vi "Tosca-Initialize IPC.vi"() -> (4 "IPC":T1, 8 "Event Registration Refnum":refnum<event-registration>, 15 "error out":errorcluster)   [LabVIEW 2020]
uses:
  Tosca-IPC.ctl
  Classes/Parameters/Parameters.lvclass
  Digital Input VIs/Tosca-DI Queue Data.ctl
  Digital Input VIs/Tosca-Input Event.ctl
  Digital Input VIs/Tosca-Input Criterion.ctl
  epl-vi-lib/Utility VIs/Type Defs/Logic State.ctl
  Typedefs/Tosca-Accumulator.ctl
  Typedefs/Tosca-State AODO.ctl
  Typedefs/Tosca-AO Runtime.ctl
  Typedefs/Tosca-DO Runtime.ctl
  epl-vi-lib/Signal Synthesis VIs/4th Generation/Classes/SignalManager/SignalManager.lvclass
  Typedefs/Tosca-Synapse Start Data.ctl
  Tosca-Message.ctl
  Tosca-Message Action.ctl
  Typedefs/Tosca-Thread Type.ctl
  Imaging VIs/Tosca-2P-Notifier Data.ctl
  Typedefs/Tosca-MATLAB Queue Data.ctl
  Visual Stim VIs/Tosca-Grating.ctl
  Visual Stim VIs/Tosca-Grating Type.ctl
  Typedefs/Tosca-File IO Notification.ctl
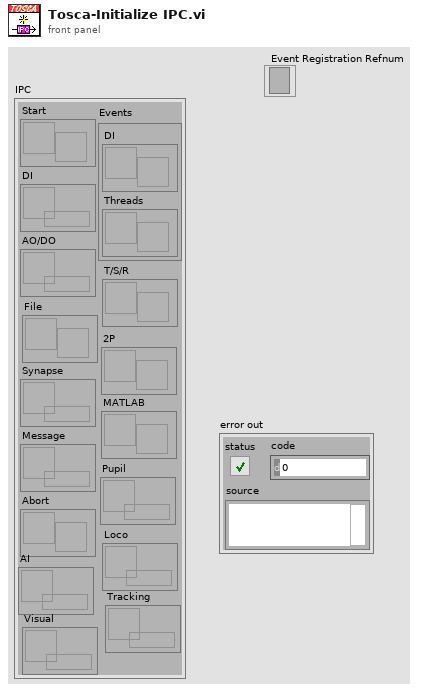
[diagram p1: front panel]
types:
  T1 = typedef "Tosca-IPC.ctl" = cluster{"Start":refnum<notifier>, "DI":refnum<queue>, "AO/DO":refnum<queue>, "Synapse":refnum<queue>, "Message":refnum<queue>, "Abort":refnum<notifier>, "Events":cluster{"DI":refnum<user-event>, "Threads ":refnum<user-event>}, "T/S/R":refnum<notifier>, "2P":refnum<notifier>, "MATLAB":refnum<notifier>, "Pupil":refnum<queue>, "Loco":refnum<queue>, "AI":refnum<queue>, "Tracking":refnum<queue>, "Visual":refnum<queue>, "File":refnum<notifier>}
  T2 = typedef "Tosca-Synapse Start Data.ctl" = cluster{"Path":path, "Codes":string, "retrieve":bool}
  T3 = typedef "Tosca-Grating.ctl" = cluster{"Type":T4, "Orientation (deg)":dbl, "Spatial frequency (cpd)":dbl, "Velocity (Hz)":dbl, "Contrast":dbl, "Background intensity":dbl, "Duration (ms)":dbl, "Phase (cycles)":dbl}
  T4 = typedef "Tosca-Grating Type.ctl" = enum16{"OFF", "Square", "Sine"}
  T5 = typedef "Tosca-MATLAB Queue Data.ctl" = cluster{"MATLAB function":path, "Datafile":path}
  T6 = typedef "Tosca-2P-Notifier Data.ctl" = cluster{"Start":bool}
  T7 = typedef "Tosca-Thread Type.ctl" = enum16{"None", "AODO", "Masker", "ET", "Imaging", "Pupil", "AI", "DI", "Camera", "TTL out", "Loco", "Visual"}
  T8 = typedef "Tosca-Message.ctl" = cluster{"Action":T9, "Time":u32, "State":i32, "Events":bool[], "Error":errorcluster}
  T9 = typedef "Tosca-Message Action.ctl" = enum16{"None", "Update", "Events", "Timeout", "Error", "Abort"}
  T10 = typedef "Tosca-File IO Notification.ctl" = cluster{"Operation":enum16{"Start", "Update", "Finish"}, "Filestem":string}
  T11 = typedef "Tosca-DI Queue Data.ctl" = cluster{"Action":enum16{"Stop", "Preview", "Run"}, "Input Events":T12[]}
  T12 = typedef "Tosca-Input Event.ctl" = cluster{"Name":string, "Criteria":T13[], "Operators":enum16{"AND", "OR"}[], "Accumulator":T15}
  T13 = typedef "Tosca-Input Criterion.ctl" = cluster{"DigInput":i32, "State":T14, "Time (ms)":i32, "Name":string}
  T14 = typedef "Logic State.ctl" = enum16{"Low", "High", "Rising", "Falling"}
  T15 = typedef "Tosca-Accumulator.ctl" = cluster{"active":bool, "N":i32, "T":dbl, "Imax":dbl, "latency":dbl}
  T16 = typedef "Tosca-State AODO.ctl" = cluster{"Name":string, "T (s)":dbl, "First AO":dbl[][], "frames/rep":i32, "finish?":bool, "Nrep":i32, "AO":T17, "DO":T18, "immediate":bool, "First DO":bool[][], "SigMan":refnum<class "SignalManager.lvclass">}
  T17 = typedef "Tosca-AO Runtime.ctl" = cluster{"Fs (Hz)":dbl, "pts/frame":i32, "pts/rep":i32, "ramp off":bool[], "fade out":dbl[][]}
  T18 = typedef "Tosca-DO Runtime.ctl" = cluster{"Fs (Hz)":dbl, "pts/frame":i32, "pts/rep":i32, "Rep":i32, "State":i32, "Trial":i32, "Frame":i32, "frOut":bool[], "Nchan":i32}
  T19 = cluster{"DI Thread State":refnum<user-event>, "Thread State":refnum<user-event>}
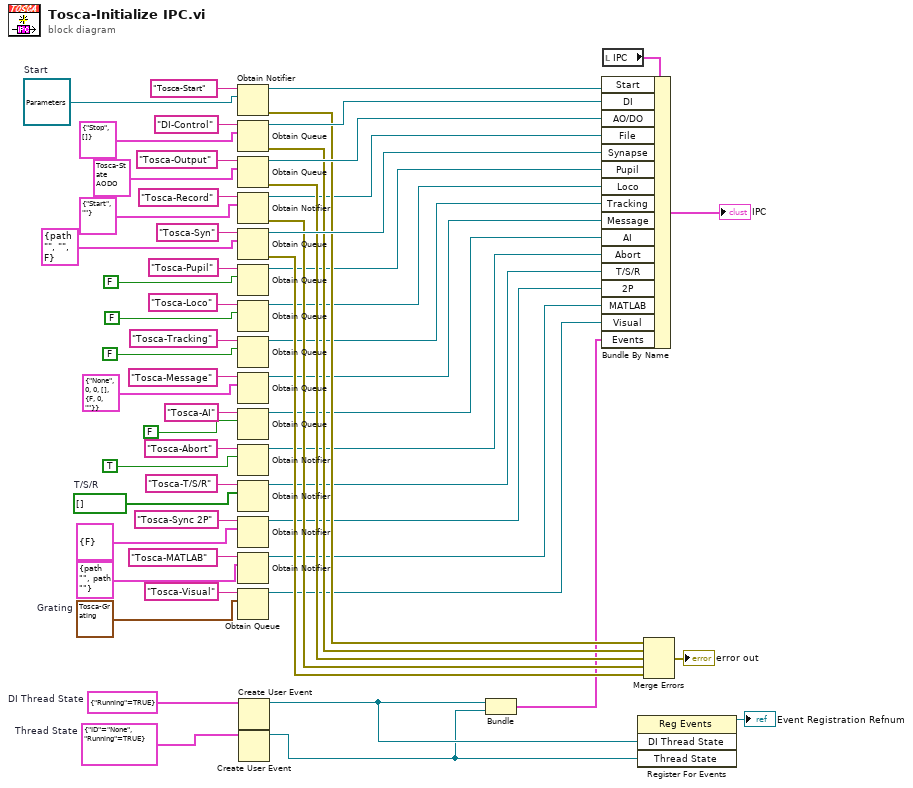
[diagram p0: block diagram]
diagram:
  w2 = refnum<class "Parameters.lvclass"> refnum  # Start
  w5 = T3 {"Type"=enum."OFF", "Orientation (deg)"=0.0, "Spatial frequency (cpd)"=0.0, "Velocity (Hz)"=0.0, "Contrast"=0.0, "Background intensity"=0.0, "Duration (ms)"=0.0, "Phase (cycles)"=0.0}  # Grating
  w26 = bool[] []  # T/S/R
  w31 = cluster{"ID":T7, "Running":bool} {"ID"=enum."None", "Running"=TRUE}  # Thread State
  w38 = cluster{"Running":bool} {"Running"=TRUE}  # DI Thread State
  n1 = Obtain Notifier(name (unnamed)="Tosca-Start" ("Start"), notification data type=w2) -> (notifier out=w53:refnum<notifier>, error out=w48:errorcluster)  [unwired: 2 in, 1 out]
  n2 = Obtain Queue(name (unnamed)="DI-Control", element data type=T11 {"Action"=enum."Stop", "Input Events"=[]} ("Cluster")) -> (queue out=w52:refnum<queue>, error out=w47:errorcluster)  [unwired: 3 in, 1 out]
  n3 = Obtain Queue(name (unnamed)="Tosca-Output", element data type=T16 {"Name"="", "T (s)"=0.0, "First AO"=[], "frames/rep"=0, "finish?"=FALSE, "Nrep"=0, "AO"={"Fs (Hz)"=0.0, "pts/frame"=0, "pts/rep"=0, "ramp off"=[], "fade out"=[]}, "DO"={"Fs (Hz)"=0.0, "pts/frame"=0, "pts/rep"=0, "Rep"=0, "State"=0, "Trial"=0, "Frame"=0, "frOut"=[], "Nchan"=0}, "immediate"=FALSE, "First DO"=[], "SigMan"=refnum} ("Output State Data")) -> (queue out=w51:refnum<queue>, error out=w46:errorcluster)  [unwired: 3 in, 1 out]
  n4 = Obtain Notifier(name (unnamed)="Tosca-Record" ("Start"), notification data type=T10 {"Operation"=enum."Start", "Filestem"=""} ("Data")) -> (notifier out=w39:refnum<notifier>, error out=w40:errorcluster)  [unwired: 2 in, 1 out]
  n5 = Obtain Queue(name (unnamed)="Tosca-Syn", element data type=T2 {"Path"=path "", "Codes"="", "retrieve"=FALSE} ("Data")) -> (queue out=w50:refnum<queue>, error out=w45:errorcluster)  [unwired: 3 in, 1 out]
  n6 = Obtain Queue(name (unnamed)="Tosca-Pupil", element data type=FALSE) -> (queue out=w16:refnum<queue>)  [unwired: 3 in, 2 out]
  n7 = Obtain Queue(name (unnamed)="Tosca-Loco", element data type=FALSE) -> (queue out=w13:refnum<queue>)  [unwired: 3 in, 2 out]
  n8 = Obtain Queue(name (unnamed)="Tosca-Tracking", element data type=FALSE) -> (queue out=w7:refnum<queue>)  [unwired: 3 in, 2 out]
  n9 = Obtain Queue(name (unnamed)="Tosca-Message", element data type=T8 {"Action"=enum."None", "Time"=0, "State"=0, "Events"=[], "Error"={"status"=FALSE, "code"=0, "source"=""}} ("Data")) -> (queue out=w35:refnum<queue>)  [unwired: 3 in, 2 out]
  n10 = Obtain Queue(name (unnamed)="Tosca-AI", element data type=FALSE) -> (queue out=w11:refnum<queue>)  [unwired: 3 in, 2 out]
  n11 = Obtain Notifier(name (unnamed)="Tosca-Abort" ("Start"), notification data type=TRUE) -> (notifier out=w32:refnum<notifier>)  [unwired: 2 in, 2 out]
  n12 = Obtain Notifier(name (unnamed)="Tosca-T/S/R" ("Start"), notification data type=w26) -> (notifier out=w25:refnum<notifier>)  [unwired: 2 in, 2 out]
  n13 = Obtain Notifier(name (unnamed)="Tosca-Sync 2P" ("Start"), notification data type=T6 {"Start"=FALSE} ("2P")) -> (notifier out=w22:refnum<notifier>)  [unwired: 2 in, 2 out]
  n14 = Obtain Notifier(name (unnamed)="Tosca-MATLAB" ("Start"), notification data type=T5 {"MATLAB function"=path "", "Datafile"=path ""} ("Data")) -> (notifier out=w19:refnum<notifier>)  [unwired: 2 in, 2 out]
  n15 = Obtain Queue(name (unnamed)="Tosca-Visual", element data type=w5) -> (queue out=w4:refnum<queue>)  [unwired: 3 in, 2 out]
  n16 = Create User Event(user event datatype=w38) -> (user event=w30:refnum<user-event>)  [unwired: 1 in, 1 out]
  n17 = Create User Event(user event datatype=w31) -> (user event=w29:refnum<user-event>)  [unwired: 1 in, 1 out]
  n18 = Bundle("DI Thread State"=w30, "Thread State"=w29) -> (w3:T19)  [unwired: 1 in]
  n19 = local read "IPC"() -> (w43:T1)
  n20 = Bundle By Name(cluster=w43, "Start"=w53, "DI"=w52, "AO/DO"=w51, "File"=w39, "Synapse"=w50, "Pupil"=w16, "Loco"=w13, "Tracking"=w7, "Message"=w35, "AI"=w11, "Abort"=w32, "T/S/R"=w25, "2P"=w22, "MATLAB"=w19, "Visual"=w4, "Events"=w3) -> (→"IPC":T1)
  n21 = register-events(w30, w29) -> (reference out=→"Event Registration Refnum":refnum<event-registration>)  [unwired: 2 in, 1 out]
  n22 = Merge Errors(w48, w47, w46, w40, w45) -> (→"error out":errorcluster)
